vi "Teleop.vi"(10 "Match Info":T1={"Autonomous Elapsed Seconds"=0.0, "TeleOp Elapsed Seconds"=0.0, "Disabled Elapsed Seconds"=0.0, "Visited Autonomous"=FALSE, "Visited TeleOp"=FALSE, "Visited Disabled"=FALSE, "Autonomous Settings"={"Autonomous Style"=enum."Independent", "VI Refnum"=refnum}}, 11 "Call Context":T2) -> ()   [LabVIEW 2013]
doc: "This VI is called for each TeleOp packet received from the DS where the robot is not disabled. It is often used to read from the joysticks and update I/O or to update setpoints for timed control loops. It should complete and return within 20 milliseconds or it may miss DS packets."
uses:
  <vilib>/Rock Robotics/WPI/DriverStation/WPI_DriverStationDerivedRobotMode.ctl
  <vilib>/Rock Robotics/WPI/DriverStation/WPI_DriverStationMatch Info.ctl
  Robot Global Data.vi
  <vilib>/Rock Robotics/WPI/Solenoid/Deprecated/WPI_SolenoidSetBool.vi
  <vilib>/Rock Robotics/WPI/Joystick/WPI_JoystickGetSetRefNum.vi
  <vilib>/Rock Robotics/WPI/RobotDrive/WPI_RobotDriveGetSetRefNum.vi
panel:
  out "Numeric 1":dbl(slide) scale=0.0..100.0
  out "Boolean 2":bool
  out "Boolean 1":bool
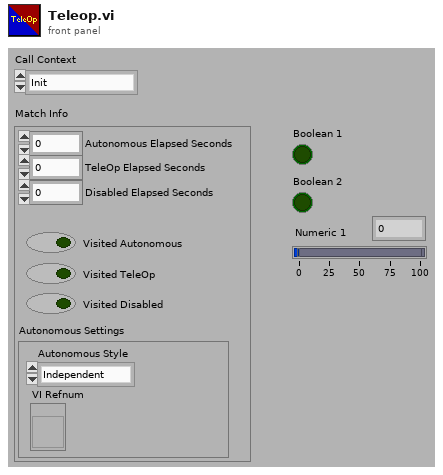
[diagram p1: front panel]
types:
  T1 = typedef "WPI_DriverStationMatch Info.ctl" = cluster{"Autonomous Elapsed Seconds":dbl, "TeleOp Elapsed Seconds":dbl, "Disabled Elapsed Seconds":dbl, "Visited Autonomous":bool, "Visited TeleOp":bool, "Visited Disabled":bool, "Autonomous Settings":cluster{"Autonomous Style":enum16{"Iterative", "Independent"}, "VI Refnum":refnum<vi>}}
  T2 = typedef "WPI_DriverStationDerivedRobotMode.ctl" = enum16{"Init", "Execute", "Stop"}
  T3 = typedef "WPI_RobotDriveDevRef.ctl" = cluster{"DevStatus":errorcluster, "Motors[]":T4[], "Square Inputs":bool, "Max Output":dbl, "Isochronous":bool}
  T4 = typedef "WPI_MotorControlDeviceRef.ctl" = cluster{"DeviceStatus":errorcluster, "Type":enum16{"PWM", "CAN"}, "PWM":cluster{"Digital Module":T5, "PWM Channel":T6, "DeadBand":T7}, "CAN":cluster{"Device Number":u8, "Control Mode":T8, "Semaphore":T9, "Max Vout":dbl}, "Invert":bool, "TransformRef":T10, "InvTransformRef":T10}
  T5 = typedef "FPGA_TypedefDigitalModule.ctl" = enum16{"Digital Module 1", "Digital Module 2"}
  T6 = typedef "FPGA_DIOPWMChannel.ctl" = enum8{"PWM 1", "PWM 2", "PWM 3", "PWM 4", "PWM 5", "PWM 6", "PWM 7", "PWM 8", "PWM 9", "PWM 10", "Invalid"}
  T7 = typedef "WPI_PWMDeadband.ctl" = cluster{"Name":string, "maxPositivePwm":i32, "minPositivePwm":i32, "centerPwm":i32, "maxNegativePwm":i32, "minNegativePwm":i32, "angularRange":u16}
  T8 = typedef "WPI_CANJaguar_ControlMode.ctl" = enum8{"Percent VBus", "Current", "Speed", "Position", "Voltage"}
  T9 = typedef "Semaphore RefNum" = refnum<k1>
  T10 = typedef "WPI_PWMTransform_ConPane.ctl" = refnum<vi>
  T11 = typedef "WPI_JoystickDevRef.ctl" = cluster{"Device":T12}
  T12 = typedef "WPI_JoystickDeviceEnum.ctl" = enum16{"USB 1", "USB 2", "USB 3", "USB 4", "Kinect 1", "Kinect 2"}
  T13 = typedef "WPI_JoystickButtonState.ctl" = cluster{"Button 1":bool, "Button 2":bool, "Button 3":bool, "Button 4":bool, "Button 5":bool, "Button 6":bool, "Button 7":bool, "Button 8":bool, "Button 9":bool, "Button 10":bool, "Button 11":bool, "Button 12":bool}
  T14 = cluster{"axis 1 (x)":dbl, "axis 2 (y)":dbl, "axis 3 (throttle)":dbl, "axis 4":dbl, "axis 5":dbl, "axis 6":dbl}
  T15 = typedef "WPI_DigitalInputDevRef.ctl" = cluster{"DevStatus":errorcluster, "DIO Channel":T16, "Digital Module":T5}
  T16 = typedef "FPGA_DIOChannel.ctl" = enum8{"DIO 1", "DIO 2", "DIO 3", "DIO 4", "DIO 5", "DIO 6", "DIO 7", "DIO 8", "DIO 9", "DIO 10", "DIO 11", "DIO 12", "DIO 13", "DIO 14", "Invalid"}
  T17 = typedef "WPI_SolenoidDevRef.ctl" = cluster{"DevStatus":errorcluster, "Solenoid Module":T18, "Forward Solenoid Channel":T19, "Reverse Solenoid Channel":T19}
  T18 = typedef "FPGA_TypedefSolenoidModule.ctl" = enum16{"Solenoid Module 1", "Solenoid Module 2"}
  T19 = typedef "WPI_SolenoidChannel.ctl" = enum8{"Solenoid 1", "Solenoid 2", "Solenoid 3", "Solenoid 4", "Solenoid 5", "Solenoid 6", "Solenoid 7", "Solenoid 8", "Invalid"}
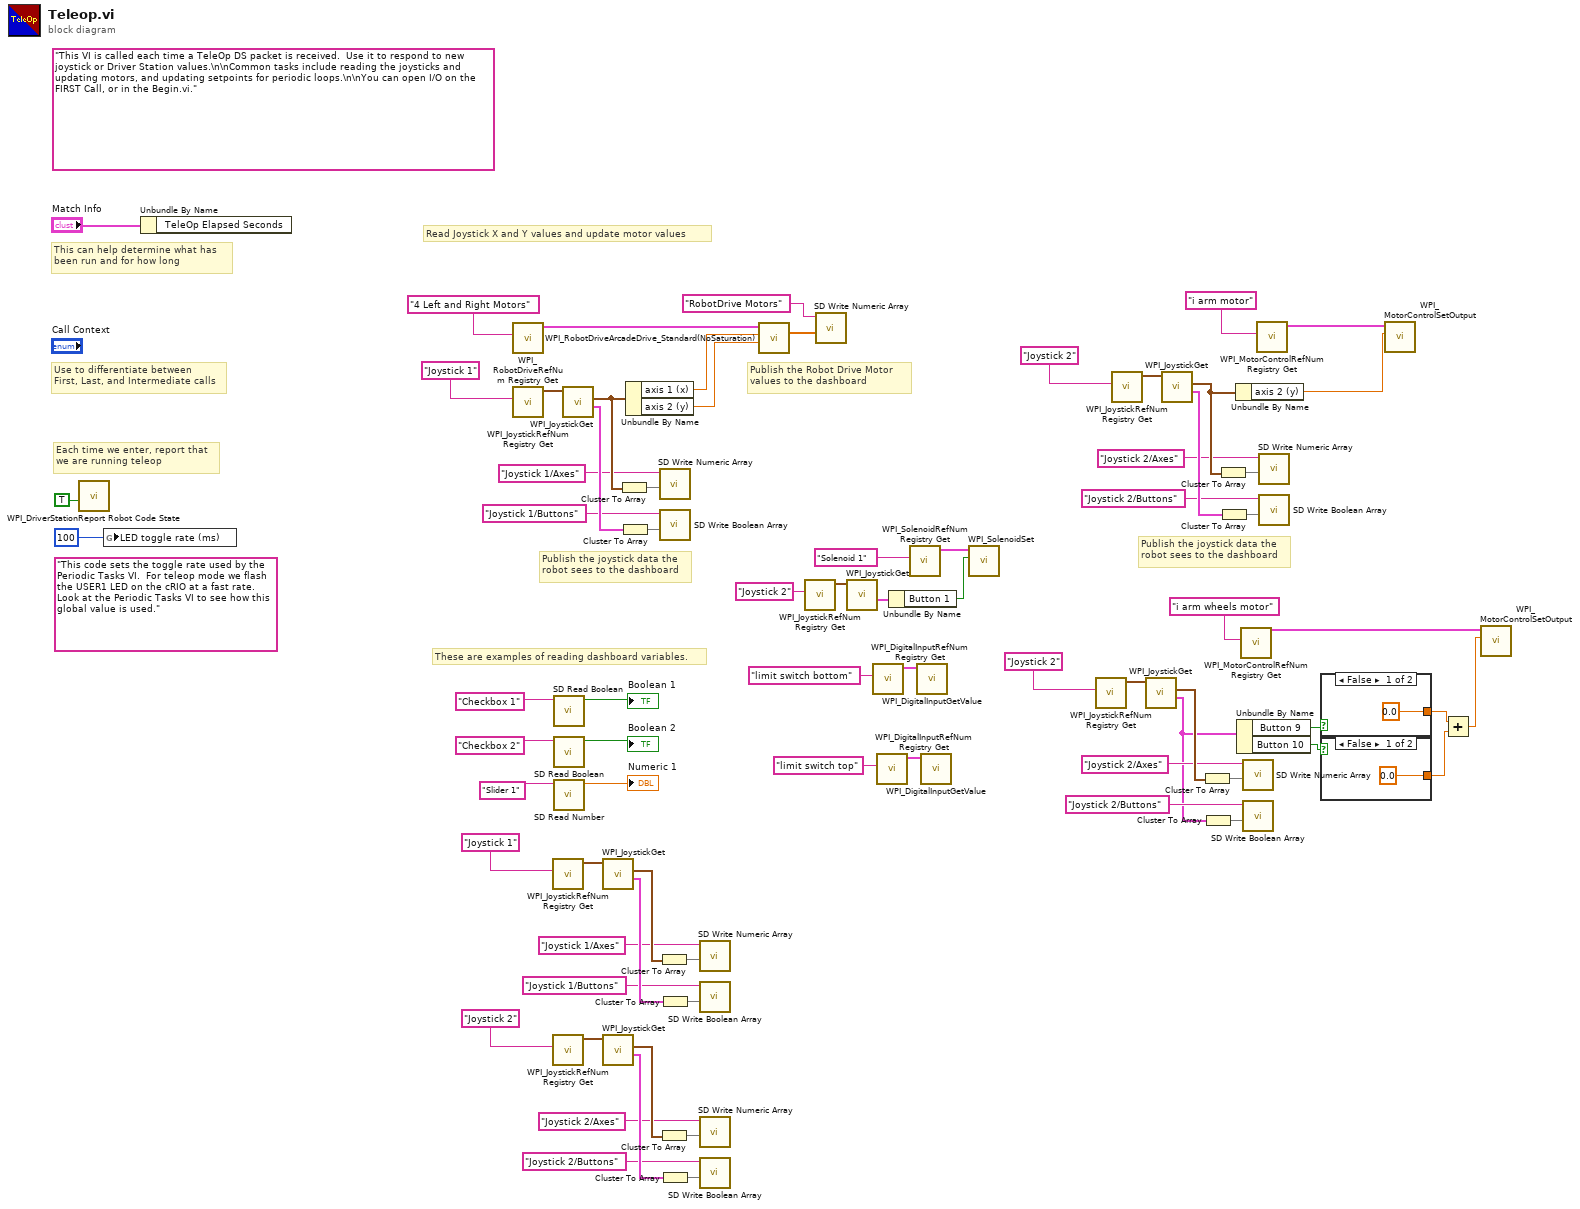
[diagram p0: block diagram]
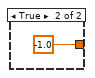
[diagram p2: hidden frame]
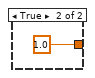
[diagram p3: hidden frame]
diagram:
  (unwired) "This code sets the toggle rate used by the Periodic Tasks VI.  For teleop mode we flash the USER1 LED on the cRIO at a fast rate.  Look at the Periodic Tasks VI to see how this global value is used."
  (unwired) "This VI is called each time a TeleOp DS packet is received.  Use it to respond to new joystick or Driver Station values.\n\nCommon tasks include reading the joysticks and updating motors, and updating setpoints for periodic loops.\n\nYou can open I/O on the FIRST Call, or in the Begin.vi."
  # "Publish the joystick data the\nrobot sees to the dashboard"
  # "These are examples of reading dashboard variables."
  # "Publish the Robot Drive Motor\nvalues to the dashboard"
  # "Publish the joystick data the\nrobot sees to the dashboard"
  # "Each time we enter, report that\nwe are running teleop"
  # "Use to differentiate between\nFirst, Last, and Intermediate calls"
  # "This can help determine what has\nbeen run and for how long"
  # "Read Joystick X and Y values and update motor values"
  n1 = call <vilib>:"WPI_DriverStationReport Robot Code State.vi"("TeleOp"=TRUE ("Autonomous")) -> ()  [unwired: 10 in, 1 out]
  n2 = global write "Robot Global Data.vi" "LED toggle rate (ms)"(u32 100 ("LED ms toggle rate")) -> ()
  n3 = Unbundle By Name("Match Info") -> ()  [unwired: 1 out]
  n4 = call <vilib>:"WPI_RobotDriveRefNum Registry Get.vi"("refnum name"="4 Left and Right Motors") -> ("RobotDriveDevRef"=w73:T3)  [unwired: 1 in, 9 out]
  n5 = call <vilib>:"WPI_JoystickRefNum Registry Get.vi"("refnum name"="Joystick 1") -> ("JoystickDevRef"=w69:T11)  [unwired: 1 in, 9 out]
  n6 = call <vilib>:"WPI_JoystickRefNum Registry Get.vi"("refnum name"="Joystick 1") -> ("JoystickDevRef"=w49:T11)  [unwired: 1 in, 9 out]
  n7 = call <vilib>:"WPI_JoystickRefNum Registry Get.vi"("refnum name"="Joystick 2") -> ("JoystickDevRef"=w39:T11)  [unwired: 1 in, 9 out]
  n8 = call <vilib>:"SD Read Boolean.vi"("Name"="Checkbox 1" ("refnum name")) -> ("Boolean"=→"Boolean 1":bool)  [unwired: 8 in, 2 out]
  n9 = call <vilib>:"SD Read Boolean.vi"("Name"="Checkbox 2" ("refnum name")) -> ("Boolean"=→"Boolean 2":bool)  [unwired: 8 in, 2 out]
  n10 = call <vilib>:"SD Read Number.vi"("Name"="Slider 1" ("refnum name")) -> ("Numeric"=→"Numeric 1":dbl)  [unwired: 8 in, 2 out]
  n11 = call <vilib>:"WPI_JoystickGet.vi"("JoystickDevRef"=w69) -> ("Buttons"=w66:T13, "Axes"=w63:T14)  [unwired: 1 in, 4 out]
  n12 = call <vilib>:"WPI_JoystickGet.vi"("JoystickDevRef"=w49) -> ("Buttons"=w48:T13, "Axes"=w45:T14)  [unwired: 1 in, 4 out]
  n13 = call <vilib>:"WPI_JoystickGet.vi"("JoystickDevRef"=w39) -> ("Buttons"=w38:T13, "Axes"=w35:T14)  [unwired: 1 in, 4 out]
  n14 = Cluster To Array(cluster=w63) -> (array=w62:dbl[])
  n15 = Cluster To Array(cluster=w66) -> (array=w65:bool[])
  n16 = Unbundle By Name(w63) -> ("axis 1 (x)"=w72:dbl, "axis 2 (y)"=w71:dbl)
  n17 = Cluster To Array(cluster=w45) -> (array=w44:dbl[])
  n18 = Cluster To Array(cluster=w35) -> (array=w34:dbl[])
  n19 = call <vilib>:"SD Write Numeric Array.vi"("Numeric Array"=w62, "Name"="Joystick 1/Axes") -> ()  [unwired: 8 in, 2 out]
  n20 = call <vilib>:"SD Write Boolean Array.vi"("Boolean Array"=w65, "Name"="Joystick 1/Buttons") -> ()  [unwired: 8 in, 2 out]
  n21 = Cluster To Array(cluster=w48) -> (array=w47:bool[])
  n22 = Cluster To Array(cluster=w38) -> (array=w37:bool[])
  n23 = call <vilib>:"SD Write Numeric Array.vi"("Numeric Array"=w44, "Name"="Joystick 1/Axes") -> ()  [unwired: 8 in, 2 out]
  n24 = call <vilib>:"SD Write Boolean Array.vi"("Boolean Array"=w47, "Name"="Joystick 1/Buttons") -> ()  [unwired: 8 in, 2 out]
  n25 = call <vilib>:"SD Write Numeric Array.vi"("Numeric Array"=w34, "Name"="Joystick 2/Axes") -> ()  [unwired: 8 in, 2 out]
  n26 = call <vilib>:"SD Write Boolean Array.vi"("Boolean Array"=w37, "Name"="Joystick 2/Buttons") -> ()  [unwired: 8 in, 2 out]
  n27 = call <vilib>:"WPI_RobotDriveArcadeDrive_Standard(NoSaturation).vi"("Y axis value"=w71, "X axis value"=w72, "RobotDriveDevRef"=w73) -> ("Motor Values"=w59:dbl[])  [unwired: 1 in, 7 out]
  n28 = call <vilib>:"WPI_JoystickRefNum Registry Get.vi"("refnum name"="Joystick 2") -> ("JoystickDevRef"=w19:T11)  [unwired: 9 in, 1 out]
  n29 = call <vilib>:"SD Write Numeric Array.vi"("Numeric Array"=w59, "Name"="RobotDrive Motors") -> ()  [unwired: 8 in, 2 out]
  n30 = call <vilib>:"WPI_JoystickGet.vi"("JoystickDevRef"=w19) -> ("Buttons"=w17:T13)  [unwired: 4 in, 2 out]
  n31 = call <vilib>:"WPI_DigitalInputRefNum Registry Get.vi"("refnum name"="limit switch bottom") -> ("DigitalInputDevRef"=w51:T15)  [unwired: 9 in, 1 out]
  n32 = call <vilib>:"WPI_DigitalInputRefNum Registry Get.vi"("refnum name"="limit switch top") -> ("DigitalInputDevRef"=w41:T15)  [unwired: 9 in, 1 out]
  n33 = Unbundle By Name(w17) -> ("Button 1"=w16:bool)
  n34 = call <vilib>:"WPI_SolenoidRefNum Registry Get.vi"("refnum name"="Solenoid 1") -> ("SolenoidDevRef"=w21:T17)  [unwired: 9 in, 1 out]
  n35 = call <vilib>:"WPI_DigitalInputGetValue.vi"("DigitalInputDevRef"=w51) -> ()  [unwired: 8 in, 3 out]
  n36 = call <vilib>:"WPI_DigitalInputGetValue.vi"("DigitalInputDevRef"=w41) -> ()  [unwired: 8 in, 3 out]
  n37 = call-poly <vilib>:"WPI_SolenoidSet.vi"("Value"=w16, "SolenoidDevRef"=w21) -> ()  [unwired: 8 in, 2 out]
  n38 = call <vilib>:"WPI_JoystickRefNum Registry Get.vi"("refnum name"="Joystick 2") -> ("JoystickDevRef"=w14:T11)  [unwired: 1 in, 9 out]
  n39 = call <vilib>:"WPI_JoystickRefNum Registry Get.vi"("refnum name"="Joystick 2") -> ("JoystickDevRef"=w31:T11)  [unwired: 1 in, 9 out]
  n40 = call <vilib>:"WPI_JoystickGet.vi"("JoystickDevRef"=w14) -> ("Buttons"=w6:T13, "Axes"=w11:T14)  [unwired: 1 in, 4 out]
  n41 = call <vilib>:"WPI_JoystickGet.vi"("JoystickDevRef"=w31) -> ("Buttons"=w30:T13, "Axes"=w27:T14)  [unwired: 1 in, 4 out]
  n42 = Cluster To Array(cluster=w11) -> (array=w10:dbl[])
  n43 = Cluster To Array(cluster=w6) -> (array=w13:bool[])
  n44 = Cluster To Array(cluster=w27) -> (array=w26:dbl[])
  n45 = Cluster To Array(cluster=w30) -> (array=w29:bool[])
  n46 = Unbundle By Name(w27) -> ("axis 2 (y)"=w22:dbl)
  n47 = Unbundle By Name(w6) -> ("Button 9"=w5:bool, "Button 10"=w4:bool)
  n48 = call <vilib>:"WPI_MotorControlRefNum Registry Get.vi"("refnum name"="i arm wheels motor") -> ("MotorControlDevRef"=w7:T4)  [unwired: 9 in, 1 out]
  n49 = call <vilib>:"SD Write Numeric Array.vi"("Numeric Array"=w10, "Name"="Joystick 2/Axes") -> ()  [unwired: 8 in, 2 out]
  n50 = call <vilib>:"SD Write Boolean Array.vi"("Boolean Array"=w13, "Name"="Joystick 2/Buttons") -> ()  [unwired: 8 in, 2 out]
  n51 = call <vilib>:"WPI_MotorControlRefNum Registry Get.vi"("refnum name"="i arm motor") -> ("MotorControlDevRef"=w23:T4)  [unwired: 9 in, 1 out]
  n52 = call <vilib>:"SD Write Numeric Array.vi"("Numeric Array"=w26, "Name"="Joystick 2/Axes") -> ()  [unwired: 8 in, 2 out]
  n53 = call <vilib>:"SD Write Boolean Array.vi"("Boolean Array"=w29, "Name"="Joystick 2/Buttons") -> ()  [unwired: 8 in, 2 out]
  n54 = case shown="False" w5 {
    tunnel: [0.0 1.0] -> w3
    frame False {
    }
    frame True {
    }
  }
  n55 = case shown="False" w4 {
    tunnel: [0.0 -1.0] -> w2
    frame False {
    }
    frame True {
    }
  }
  n56 = call <vilib>:"WPI_MotorControlSetOutput.vi"("Output"=w22, "MotorControlDevRef"=w23) -> ()  [unwired: 7 in, 3 out]
  n57 = Add(x=w3, y=w2) -> (x+y=w1:dbl)
  n58 = call <vilib>:"WPI_MotorControlSetOutput.vi"("Output"=w1, "MotorControlDevRef"=w7) -> ()  [unwired: 7 in, 3 out]
